vi "Launch Valve Actor.vi"(0 "Caller Actor in":refnum<class "Actor.lvclass">, 1 "Name":string, 2 "Start Action (Open)":T1, 3 "DedicatedEnQrs":refnum<queue>, 5 "Interlock Chain":refnum<class "Interlock Chain.lvclass">, 7 "Valve in":refnum<class "Valve.lvclass">, 9 "SHV Aliases":refnum<k21>[](array[refnum]), 11 "error in (no error)":errorcluster, 12 "SHV":refnum<k21>[](array[refnum]), 13 "StateQ":refnum<queue>, 14 "Stop Action (Close)":T1=enum."Close") -> (4 "Caller-To-Actor Enqueuer":refnum<class "Message Enqueuer.lvclass">, 15 "error out":errorcluster)   [LabVIEW 2015, in "cRIO-Carbondioxide.lvlib" / "CO2-Actor.lvlib" / "Valve.lvclass"]
uses:
  Valve.lvclass
  <vilib>/ActorFramework/Actor/Actor.lvclass
  Interlocks/Interlock Chain/Interlock Chain.lvclass
  <vilib>/ActorFramework/Message Enqueuer/Message Enqueuer.lvclass
  Action.ctl
  Controls/Dedicated Enqueuers.ctl
  CO2 Actor/CO2 Actor.lvclass
  Valve.lvclass/Valve.ctl
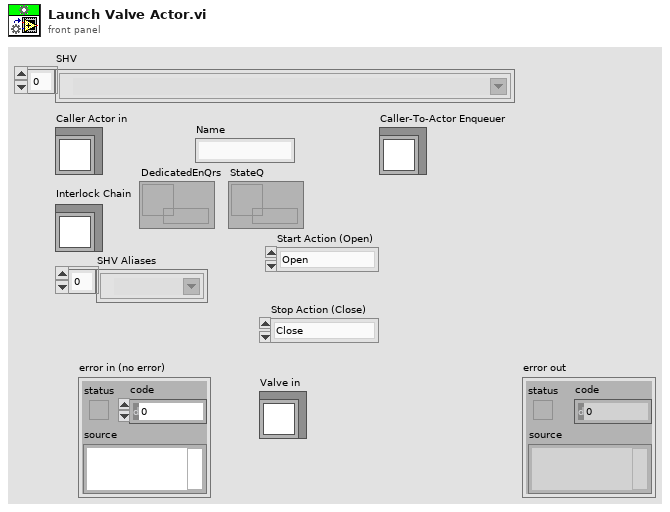
[diagram p1: front panel]
types:
  T1 = typedef "Action.ctl" = enum16{"Open", "Close", "None"}
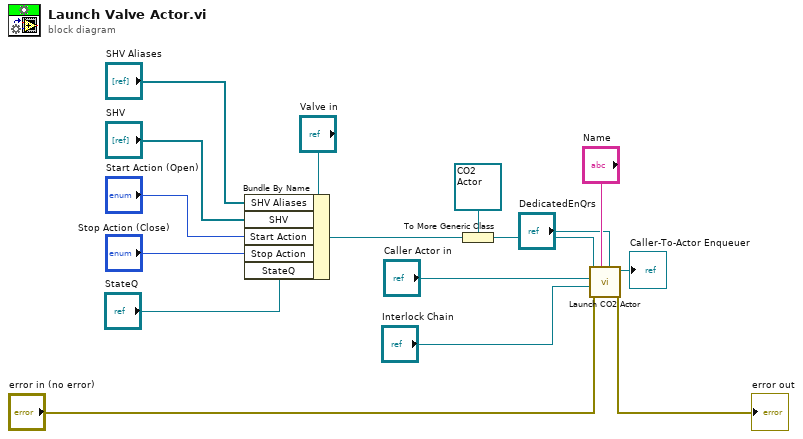
[diagram p0: block diagram]
diagram:
  n1 = Bundle By Name(cluster="Valve in", "SHV Aliases"="SHV Aliases", "SHV"="SHV", "Start Action"="Start Action (Open)", "Stop Action"="Stop Action (Close)", "StateQ"="StateQ") -> (w7:refnum<class "Valve.lvclass">)
  n2 = To More Generic Class(target class=refnum<class "CO2 Actor.lvclass"> refnum ("CO2 Actor in"), reference=w7) -> (generic class reference=w5:refnum<class "CO2 Actor.lvclass">)
  n3 = call "Launch CO2 Actor.vi"("DedicatedEnQrs"="DedicatedEnQrs", "Name"="Name", "error in (no error)"="error in (no error)", "Interlock Chain"="Interlock Chain", "Caller Actor in"="Caller Actor in", "CO2 Actor in"=w5) -> ("error out"=→"error out":errorcluster, "Caller-To-Actor Enqueuer"=→"Caller-To-Actor Enqueuer":refnum<class "Message Enqueuer.lvclass">)  [unwired: 4 in]
